vi "Door Booleans2.vi"() -> ()   [LabVIEW 2026]
uses:
  user32.dll
panel:
  out "String":string
  in  "Close":bool
  out "magnalock-map-e":bool
  out "magnalock-map-a":bool
  out "magnalock-map-b":bool
  out "magnalock-map-d":bool
  out "magnalock-map-c":bool
  out "door-map-d":bool caption="Door D"
  out "door-map-c":bool caption="Door C"
  out "door-map-b":bool caption="Door B"
  out "door-map-e":bool caption="Door E"
  out "door-map-a":bool caption="Door A"
  in  "header":bool
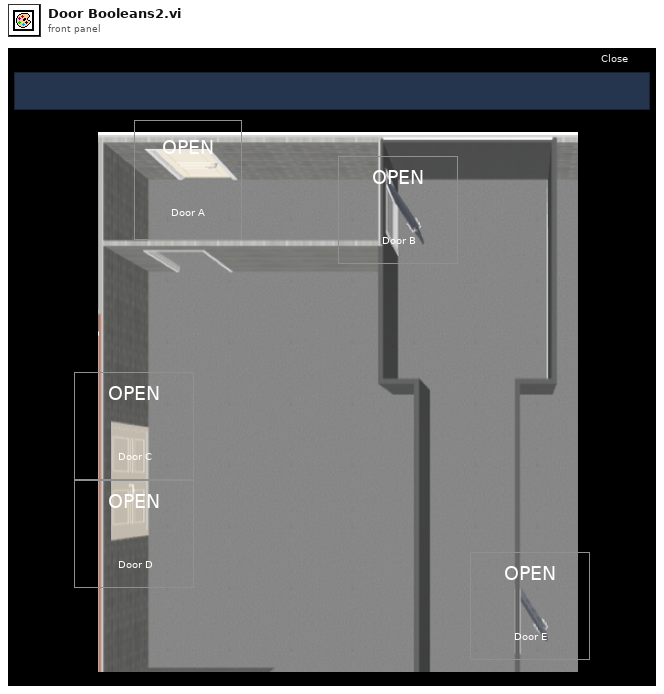
[diagram p1: front panel]
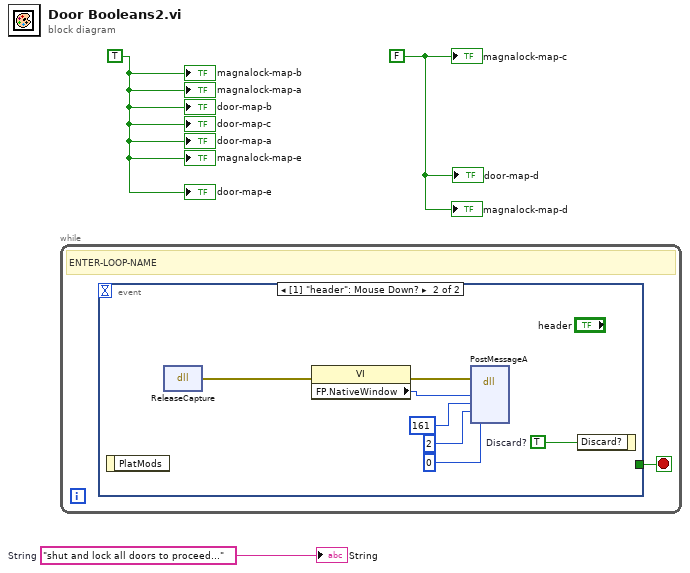
[diagram p0: block diagram]
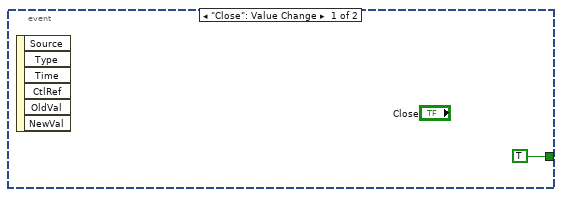
[diagram p2: hidden frame]
diagram:
  w1 = TRUE
  w2 = FALSE
  w3 = "shut and lock all doors to proceed..."  # String
  n1 = while {
    stop <- w4 stop-if-true
    # "ENTER-LOOP-NAME"
    n2 = event shown="[1] \"header\": Mouse Down?" {
      selector: _ -> [_ _]
      dyn-events: _ -> [_ _]
      timeout: _ -> [_ _]
      tunnel: [TRUE _] -> w4
      event "Close": Value Change {
        n3 = event-data() -> ()  [unwired: 1 in, 6 out]
      }
      event "header": Mouse Down? {
        w12 = TRUE  # Discard?
        n4 = event-data() -> ()  [unwired: 1 in, 1 out]
        n5 = dll-call lib="user32.dll" fn="ReleaseCapture"() -> (error out=w8:errorcluster)  [unwired: 4 in, 1 out]
        n6 = property class="VI"(error in=w8) -> (error out=w7:errorcluster, "FP.NativeWindow"=w6:u64)  [unwired: 1 in, 1 out]
        n7 = dll-call lib="user32.dll" fn="PostMessageA"(error in=w7, "hWnd"=w6, "Msg"=161, "wParam"=2, "lParam"=0) -> ()  [unwired: 7 in, 2 out]
        n8 = event-data("Discard?"=w12) -> ()  [unwired: 1 in, 1 out]
      }
    }
  }
  "door-map-a" <- w1
  "door-map-e" <- w1
  "door-map-b" <- w1
  "door-map-c" <- w1
  "door-map-d" <- w2
  "magnalock-map-c" <- w2
  "magnalock-map-d" <- w2
  "magnalock-map-b" <- w1
  "magnalock-map-a" <- w1
  "magnalock-map-e" <- w1
  "String" <- w3
